vi "Dispense Function (SubVI).vi"(0 "Signals IN":T3={"Dispense"=FALSE, "Fill"=FALSE, "Spray"=FALSE, "Drain"=TRUE, "Complete"=FALSE, "Fill Error"=FALSE, "Dispense Error"=FALSE, "Fill Timeout"=FALSE, "Dispense Timeout"=FALSE}, 1 "Values IN":T4 {"Drain Time (s)" format="%.2f"; "Drain Rate (g/sec)" format="%.2f"; "Time Elapsed (s)" format="%.2f"; "Time Target (s)" format="%.2f"; "Dynamic Setpoint (g)" format="%.2f"; "Static Setpoint (g)" format="%.2f"; "Grams to Setpoint" format="%.2f"; "Adjusted Mass (g)" format="%.2f"; "Dispense Rate (g/sec)" format="%.2f"; "Fill Mass (g)" format="%.2f"; "Fill Rate (g/sec)" format="%.2f"}, 2 "Measured Mass (g)":dbl, 3 "Main Concentration Setpoint (%)":dbl, 4 "Product Weight (g)":dbl, 5 "Settings":T2={"ON Settings"={"Enable Dynamic Setpoint?"=TRUE, "Enable Dynamic Dispense Time?"=TRUE, "Enable Drain Rate Functions"=TRUE, "Dispense Sample Time (s)"=0.5, "Dispense Slope Ave"=0, "ON Timeout (sec)"=600.0, "1st Setpoint (% of Target)"=0.0, "2nd Setpoint (% of Target)"=0.0, "3rd Setpoint (% of Target)"=0.0, "Measure Dispense Delay (sec)"=0.0, "Settle Slope Sample Time (s)"=0.0}, "OFF Settings"={"Drain Sample Time (s)"=0.5, "Drain Rate Ave Size"=5, "Drain Rate Limits (± g/sec)"=10.0, "Level Slope Range (± g/sec)"=0.25, "OFF Timeout (sec)"=0.0, "Near SP Slope Level (± g/sec)"=0.01, "Near Setpoint Threshold (%)"=95.0}, "Overshoot Settings"={"Time Limit (s)"=60.0, "Container MAX (g)"=1500.0, "Max FILL Slope (+/- g/sec)"=10.0, "% Overshot to Enable (>)"=0.25}, "FILL Timeout (s)"=300.0, "Full Settle Time (s)"=20.0, "Pre-Hydrate \nSpray Time (s)"=10.0, "Pre-Hydrate \nWait Time (s)"=30.0}, 9 "Main Case Change?":bool) -> (14 "Signals OUT":T3={"Dispense"=FALSE, "Fill"=FALSE, "Spray"=FALSE, "Drain"=TRUE, "Complete"=FALSE, "Fill Error"=FALSE, "Dispense Error"=FALSE, "Fill Timeout"=FALSE, "Dispense Timeout"=FALSE}, 15 "Values OUT":T4 {"Drain Time (s)" format="%.2f"; "Drain Rate (g/sec)" format="%.2f"; "Time Elapsed (s)" format="%.2f"; "Time Target (s)" format="%.2f"; "Dynamic Setpoint (g)" format="%.2f"; "Static Setpoint (g)" format="%.2f"; "Grams to Setpoint" format="%.2f"; "Adjusted Mass (g)" format="%.2f"; "Dispense Rate (g/sec)" format="%.2f"; "Fill Mass (g)" format="%.2f"; "Fill Rate (g/sec)" format="%.2f"}, 17 "Product Values":T1, 18 "Hydration (g)":dbl, 19 "Dispense Complete?":bool)   [LabVIEW 2012]
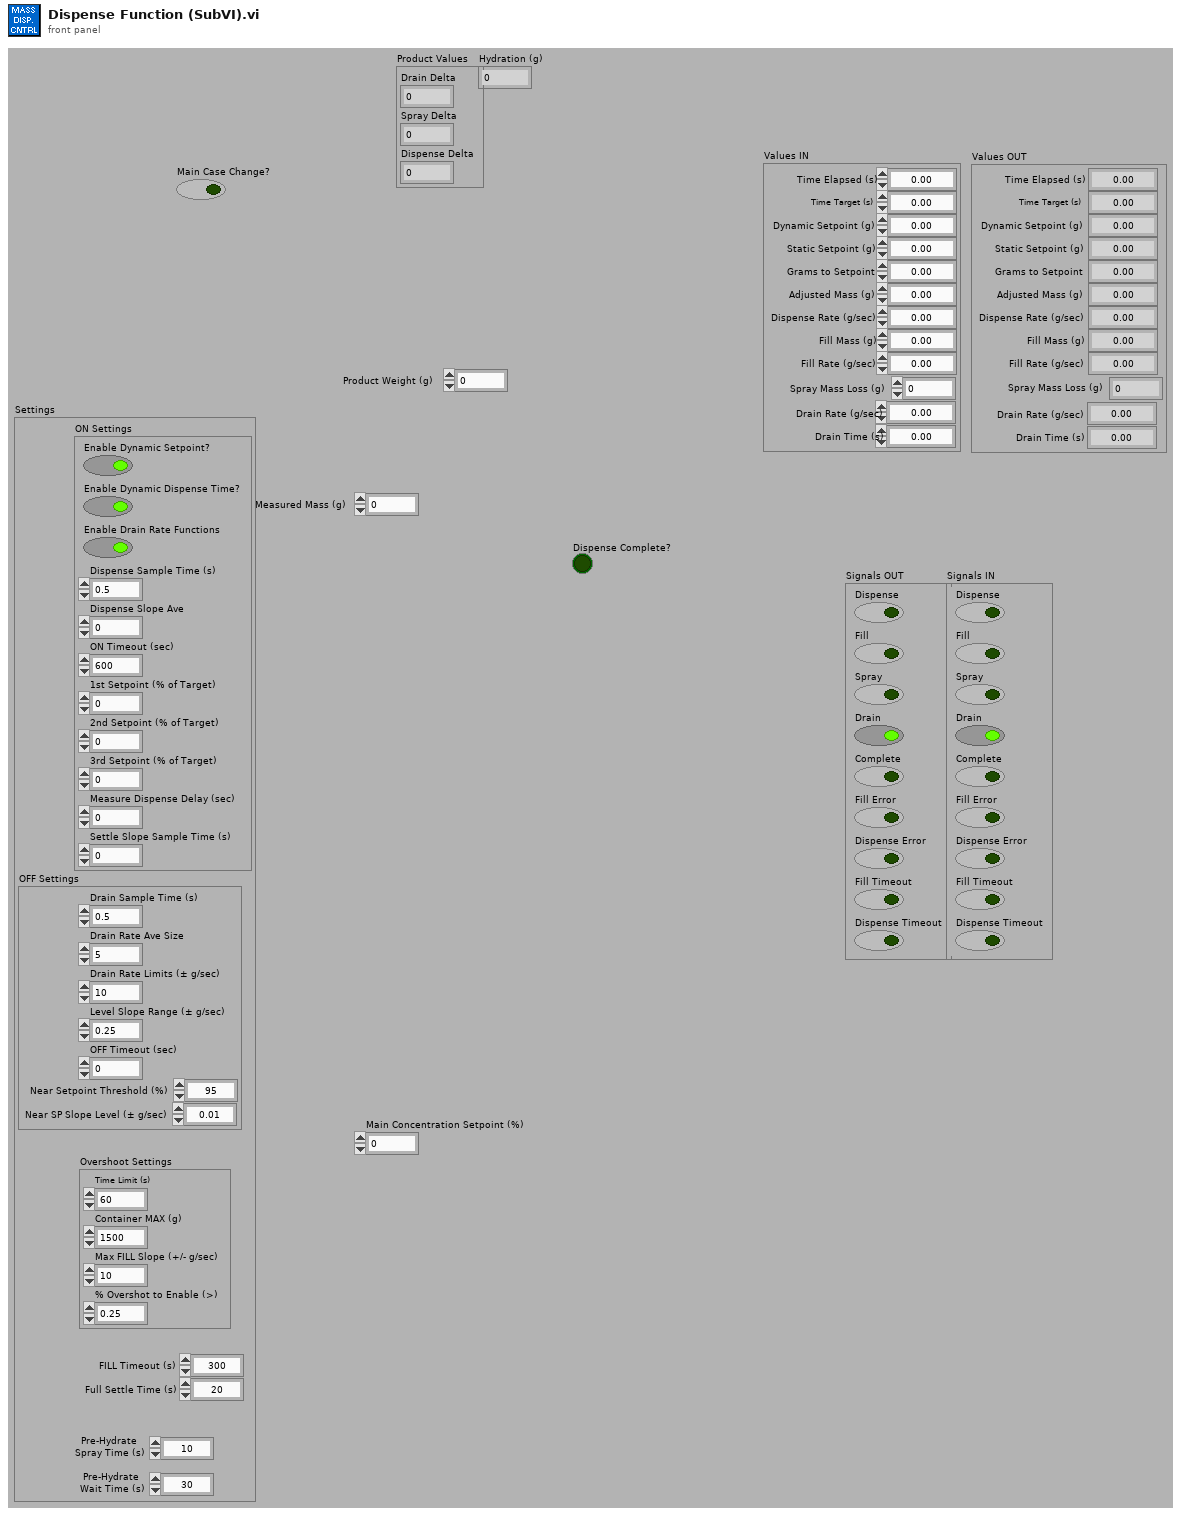
[diagram p1: front panel]
types:
  T1 = cluster{"Drain Delta":dbl, "Spray Delta":dbl, "Dispense Delta":dbl}
  T2 = cluster{"ON Settings":cluster{"Enable Dynamic Setpoint?":bool, "Enable Dynamic Dispense Time?":bool, "Enable Drain Rate Functions":bool, "Dispense Sample Time (s)":dbl, "Dispense Slope Ave":i32, "ON Timeout (sec)":dbl, "1st Setpoint (% of Target)":dbl, "2nd Setpoint (% of Target)":dbl, "3rd Setpoint (% of Target)":dbl, "Measure Dispense Delay (sec)":dbl, "Settle Slope Sample Time (s)":dbl}, "OFF Settings":cluster{"Drain Sample Time (s)":dbl, "Drain Rate Ave Size":i32, "Drain Rate Limits (± g/sec)":dbl, "Level Slope Range (± g/sec)":dbl, "OFF Timeout (sec)":dbl, "Near SP Slope Level (± g/sec)":dbl, "Near Setpoint Threshold (%)":dbl}, "Overshoot Settings":cluster{"Time Limit (s)":dbl, "Container MAX (g)":dbl, "Max FILL Slope (+/- g/sec)":dbl, "% Overshot to Enable (>)":dbl}, "FILL Timeout (s)":dbl, "Full Settle Time (s)":dbl, "Pre-Hydrate \nSpray Time (s)":dbl, "Pre-Hydrate \nWait Time (s)":dbl}
  T3 = cluster{"Dispense":bool, "Fill":bool, "Spray":bool, "Drain":bool, "Complete":bool, "Fill Error":bool, "Dispense Error":bool, "Fill Timeout":bool, "Dispense Timeout":bool}
  T4 = cluster{"Time Elapsed (s)":dbl, "Time Target (s)":dbl, "Dynamic Setpoint (g)":dbl, "Static Setpoint (g)":dbl, "Grams to Setpoint":dbl, "Adjusted Mass (g)":dbl, "Dispense Rate (g/sec)":dbl, "Fill Mass (g)":dbl, "Fill Rate (g/sec)":dbl, "Spray Mass Loss (g)":dbl, "Drain Rate (g/sec)":dbl, "Drain Time (s)":dbl}
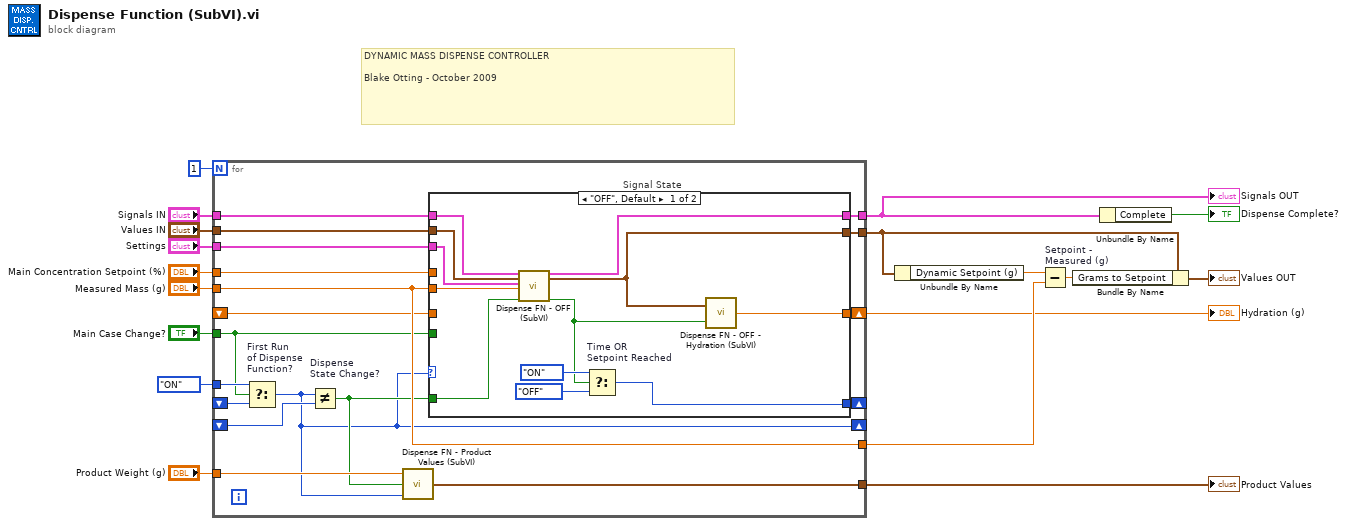
[diagram p0: block diagram]
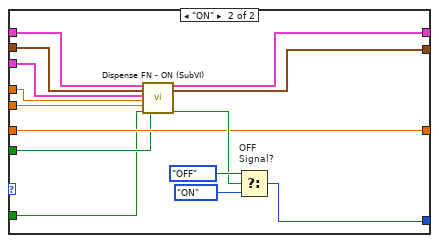
[diagram p2: hidden frame]
diagram:
  # "DYNAMIC MASS DISPENSE CONTROLLER\n\nBlake Otting - October 2009"
  n1 = for {
    N: 1 -> [_]
    tunnel: "Measured Mass (g)" -> [w30]
    tunnel: "Settings" -> [w36]
    shift-right: [w34] -> _
    shift-left: _ -> [w26]
    tunnel: "Main Concentration Setpoint (%)" -> [w35]
    tunnel: "Values IN" -> [w33]
    tunnel: [w32] -> w8
    tunnel: [w31] -> w11
    tunnel: "Signals IN" -> [w19]
    tunnel: [w30] -> w9
    shift-right: [w29] -> w5
    shift-left: _ -> [w28]
    tunnel: enum16{"OFF", "ON"}."ON" ("Signal State 2") -> [w27]
    tunnel: "Main Case Change?" -> [w21]
    tunnel: [w25] -> w2
    tunnel: "Product Weight (g)" -> [w24]
    shift-right: [w20] -> _
    shift-left: _ -> [w23]
    n2 = Select "First Run\nof Dispense\nFunction?"(t=w27, s=w21, f=w26) -> (s? t:f=w20:enum16{"OFF", "ON"})
    n3 = Not Equal? "Dispense\nState Change?"(x=w20, y=w23) -> (x != y?=w22:bool)
    n4 = call "Dispense FN - Product Values (SubVI).vi"("State Input"=w20, "Dispense State Change?"=w22, "Product Weight (g)"=w24) -> ("Product Values"=w25:T1)
    n5 = case "Signal State" shown="\"OFF\", Default" w20 {
      tunnel: w30 -> [w45 w52]
      tunnel: w36 -> [w37 w49]
      tunnel: [w47 w60] -> w34
      tunnel: w35 -> [_ w50]
      tunnel: w33 -> [w44 w55]
      tunnel: w19 -> [w43 w57]
      tunnel: [w41 w56] -> w32
      tunnel: [w42 w58] -> w31
      tunnel: [w39 w54] -> w29
      tunnel: w28 -> [_ w54]
      tunnel: w22 -> [w38 w51]
      tunnel: w21 -> [_ w53]
      frame "OFF", Default {
        n6 = call "Dispense FN - OFF (SubVI).vi"("Signals IN"=w43, "Values IN"=w44, "Settings"=w37, "Measured Mass (g)"=w45, "State Change?"=w38) -> ("Signals OUT"=w42:T3, "Values OUT"=w41:T4, "ON Signal"=w40:bool)  [unwired: 2 in, 10 out]
        n7 = Select "Time OR\nSetpoint Reached"(t=enum16{"OFF", "ON"}."ON" ("Mode (Read)"), s=w40, f=enum16{"OFF", "ON"}."OFF" ("Mode (Read)")) -> (s? t:f=w47:enum16{"OFF", "ON"})
        n8 = call "Dispense FN - OFF - Hydration (SubVI).vi"("ON Signal"=w40, "Values"=w41) -> ("Hydration (g)"=w39:dbl)
      }
      frame "ON" {
        n9 = call "Dispense FN - ON (SubVI).vi"("Signals IN"=w57, "Values IN"=w55, "Settings"=w49, "Main Concentration Setpoint (%)"=w50, "Measured Mass (g)"=w52, "State Change?"=w51, "Main Case Change?"=w53) -> ("Signals OUT"=w58:T3, "Values OUT"=w56:T4, "OFF Signal"=w59:bool)  [unwired: 1 in, 9 out]
        n10 = Select "OFF\nSignal?"(t=enum16{"OFF", "ON"}."OFF" ("Signal State 2"), s=w59, f=enum16{"OFF", "ON"}."ON" ("Signal State 2")) -> (s? t:f=w60:enum16{"OFF", "ON"})
      }
    }
  }
  "Signals OUT" <- w11
  "Product Values" <- w2
  "Hydration (g)" <- w5
  n11 = Unbundle By Name(w8) -> ("Dynamic Setpoint (g)"=w7:dbl)
  n12 = Subtract "Setpoint -\nMeasured (g)"(x=w7, y=w9) -> (x-y=w6:dbl)
  n13 = Bundle By Name(cluster=w8, "Grams to Setpoint"=w6) -> (→"Values OUT":T4)
  n14 = Unbundle By Name(w11) -> ("Complete"=→"Dispense Complete?":bool)
